vi "MemBlockInit(Path).vi"(8 "error in (no error)":errorcluster caption="错误输入（无错误）", 11 "内存块标签列表":cluster{"Name":string, "Default Value":path}[](array[cluster])) -> (0 "error out":errorcluster caption="错误输出")   [LabVIEW 2012, in "MemBlock.lvlib"]
uses:
  MemBlock.lvlib
  MemBlock/MemBlock(Path).vi
  MemBlockTag/MemBlockTagList(Path).vi
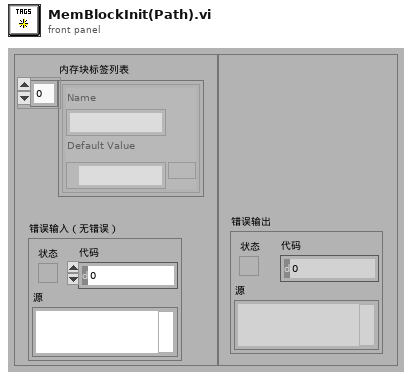
[diagram p1: front panel]
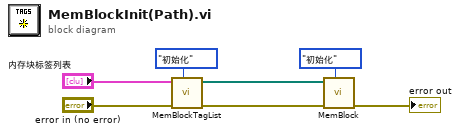
[diagram p0: block diagram]
diagram:
  n1 = call-poly "MemBlockTagList.vi"("方法"=enum16{"初始化", "获取索引"}."初始化", "error in (no error)"="error in (no error)", "内存块标签列表"="内存块标签列表") -> ("error out"=w4:errorcluster, "默认值"=w1:path[])  [unwired: 6 in, 1 out]
  n2 = call-poly "MemBlock.vi"("方法"=enum16{"初始化", "读取", "读取全部", "写入"}."初始化", "error in (no error)"=w4, "默认值"=w1) -> ("error out"=→"error out":errorcluster)  [unwired: 6 in, 2 out]
